vi "FormulaGeneral.vi"() -> ()   [LabVIEW 2018]
panel:
  out "X2":dbl
  out "X1":dbl
  in  "C":dbl
  in  "B":dbl
  in  "A":dbl
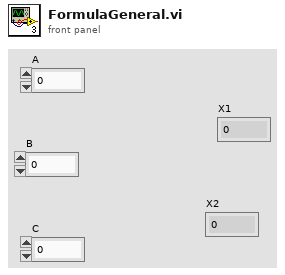
[diagram p1: front panel]
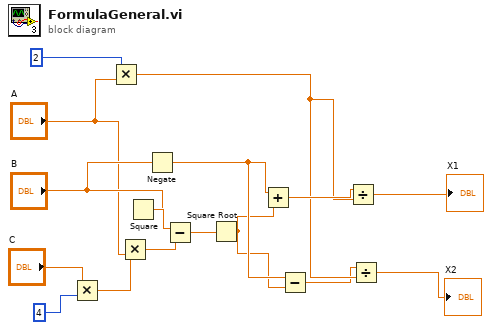
[diagram p0: block diagram]
diagram:
  n1 = Multiply(x="C", y=4) -> (x*y=w14:dbl)
  n2 = Multiply(x=2, y="A") -> (x*y=w2:dbl)
  n3 = Multiply(x=w14, y="A") -> (x*y=w12:dbl)
  n4 = Square(x="B") -> (x^2=w13:dbl)
  n5 = Negate(x="B") -> (-x=w9:dbl)
  n6 = Subtract(x=w13, y=w12) -> (x-y=w11:dbl)
  n7 = Square Root(x=w11) -> (sqrt(x)=w8:dbl)
  n8 = Add(x=w9, y=w8) -> (x+y=w3:dbl)
  n9 = Subtract(x=w9, y=w8) -> (x-y=w1:dbl)
  n10 = Divide(x=w3, y=w2) -> (x/y=→"X1":dbl)
  n11 = Divide(x=w1, y=w2) -> (x/y=→"X2":dbl)
